vi "Pre Launch Init.vi"(11 "IModel in":refnum<class "IModel.lvclass">) -> (0 "error out":errorcluster, 3 "IModel out":refnum<class "IModel.lvclass">)   [LabVIEW 2020, in "MVA Framework.lvlib" / "IModel.lvlib" / "IModel.lvclass"]
doc: "(<B>Filename</B>: Actor Framework.lvlib:Actor.lvclass:Pre Launch Init.vi)\n\nDefines behavior that occurs after the Launch Nested Actor method is invoked but before the actor's Actor Core method begins running.\n\nBy default, this method does nothing. A descendant class may override it to define behavior."
uses:
  IModel.lvclass
  C:/Program Files/National Instruments/LabVIEW 2020/vi.lib/ActorFramework/Actor/Actor.lvclass
  <vilib>/ActorFramework/Actor/Actor.lvclass/Actor.ctl
  <vilib>/ActorFramework/Message Enqueuer/Message Enqueuer.lvclass/Message Enqueuer.ctl
  IModel.lvclass/IModel.ctl
  <vilib>/ActorFramework/Message Enqueuer/Init from Existing Queue.vi
  IObserver/IObserver/IObserver.lvclass
  <vilib>/ActorFramework/Message Enqueuer/Message Enqueuer.lvclass
  IModel Messages/Auto-Launch Models Msg/Auto-Launch Models Msg.lvclass
  <vilib>/ActorFramework/Actor/Actor.lvclass
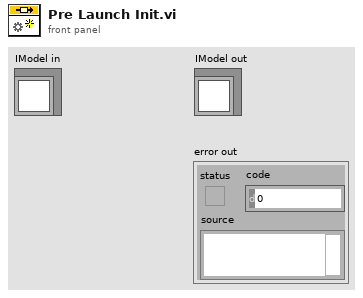
[diagram p1: front panel]
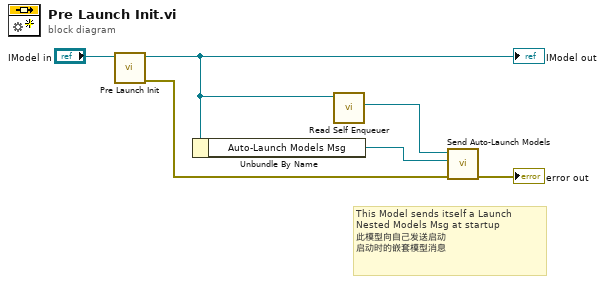
[diagram p0: block diagram]
diagram:
  # "This Model sends itself a Launch\nNested Models Msg at startup\n此模型向自己发送启动\n启动时的嵌套模型消息"
  n1 = call-parent "Pre Launch Init.vi"("IObserver in"="IModel in") -> ("error out"=w4:errorcluster, "IObserver out"=w2:refnum<class "IModel.lvclass">)  [unwired: 9 in]
  "IModel out" <- w2
  n2 = Unbundle By Name(w2) -> ("Auto-Launch Models Msg"=w1:refnum<class "Auto-Launch Models Msg.lvclass">)
  n3 = call <vilib>:"Read Self Enqueuer.vi"("Actor"=w2) -> ("Self Enqueuer"=w5:refnum<class "Message Enqueuer.lvclass">)  [unwired: 10 in]
  n4 = call-dynamic "Send Auto-Launch Models.vi"("error in (no error)"=w4, "Launch Nested Models Msg"=w1, "Message Enqueuer"=w5) -> ("error out"=→"error out":errorcluster)  [unwired: 7 in, 1 out]
